vi "get_ramp_from_wavefrom.vi"(11 "waveform in":waveform(dbl)) -> (3 "ramp pattern out":dbl[](array[numeric]))   [LabVIEW 2020]
uses:
  <vilib>/Analysis/1siggen.llb/Ramp Pattern by Samples.vi
  <vilib>/Waveform/WDTOps.llb/WDT Waveform Duration DBL.vi
  <vilib>/Analysis/NI_AALBase.lvlib
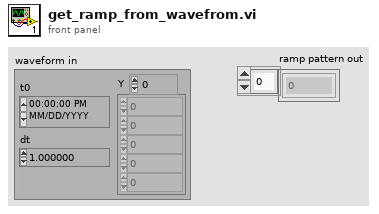
[diagram p1: front panel]
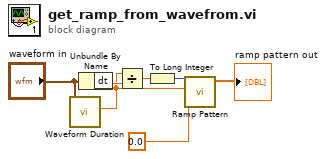
[diagram p0: block diagram]
diagram:
  n1 = call-poly <vilib>:"Waveform Duration.vi"("waveform in"="waveform in") -> ("duration"=w2:dbl)  [unwired: 8 in, 2 out]
  n2 = Unbundle By Name("waveform in") -> ("dt"=w3:dbl)
  n3 = Divide(x=w2, y=w3) -> (x/y=w5:dbl)
  n4 = To Long Integer(number=w5) -> (32bit integer=w4:i32)
  n5 = call-poly <vilib>:"Ramp Pattern.vi"("start"=0.0, "end"=w2, "samples"=w4) -> ("Ramp Pattern"=→"ramp pattern out":dbl[])  [unwired: 7 in, 1 out]
